vi "Get Attribute Name and Parent ID from Tag.vi"(8 "error in (no error)":errorcluster, 10 "Tag":string, 11 "Linked List in":refnum<class "Linked List.lvclass">) -> (0 "error out":errorcluster, 1 "Attribute Name":string, 2 "Linked List ID":string, 3 "Linked List out":refnum<class "Linked List.lvclass">)   [LabVIEW 2020, in "Linked Lists.lvlib" / "Linked List.lvclass"]
uses:
  <vilib>/gpm_packages/@cs/linked-list/Source/Linked List/Linked List/Linked List.lvclass
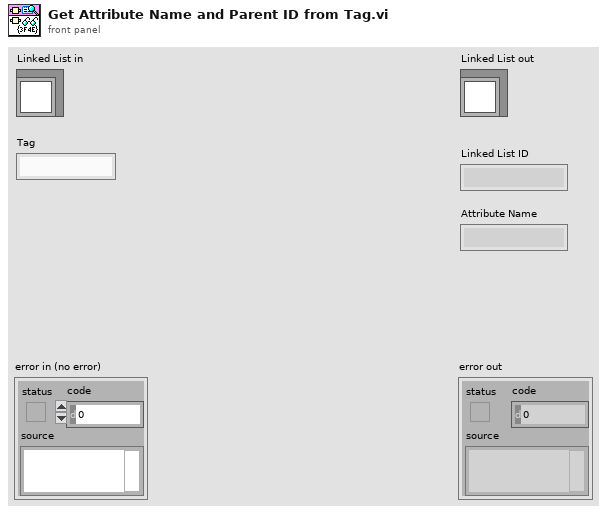
[diagram p1: front panel]
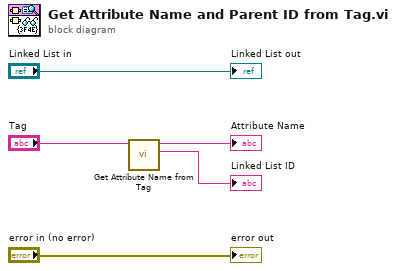
[diagram p0: block diagram]
diagram:
  n1 = call <vilib>:"Get Attribute Name from Tag.vi"("Tag"="Tag") -> ("Linked List ID"=→"Linked List ID":string, "Attribute Name"=→"Attribute Name":string)  [unwired: 8 in, 1 out]
  "error out" <- "error in (no error)"
  "Linked List out" <- "Linked List in"
